vi "ACP Configure Offset Channel.vi"(7 "Selector String":string, 8 "error in (no error)":errorcluster, 10 "ACP Offset Channel Configuration":T1=[{"Offset Frequency"={"Frequency (Hz)"=20000000.0, "Sideband"=2}, "Offset Power Reference"={"Specific Index"=0, "Carrier"=0}, "Integration Bandwidth (Hz)"=18000000.0, "Relative Attenuation (dB)"=0.0, "RRC Filter"={"Alpha"=0.22, "Enabled"=0}, "Enabled"=1}, {"Offset Frequency"={"Frequency (Hz)"=12500000.0, "Sideband"=2}, "Offset Power Reference"={"Specific Index"=0, "Carrier"=0}, "Integration Bandwidth (Hz)"=3840000.0, "Relative Attenuation (dB)"=0.0, "RRC Filter"={"Alpha"=0.22, "Enabled"=0}, "Enabled"=1}, {"Offset Frequency"={"Frequency (Hz)"=17500000.0, "Sideband"=2}, "Offset Power Reference"={"Specific Index"=0, "Carrier"=0}, "Integration Bandwidth (Hz)"=3840000.0, "Relative Attenuation (dB)"=0.0, "RRC Filter"={"Alpha"=0.22, "Enabled"=0}, "Enabled"=1}] {"Enabled" items=["False", "True"]; "Offset Power Reference"."Carrier" items=["Closest", "Highest", "Composite", "Specific"]; "RRC Filter"."Enabled" items=["False", "True"]; "RRC Filter"."Alpha" format="%.3g"; "Relative Attenuation (dB)" format="%.2f"; "Integration Bandwidth (Hz)" format="%.3p"; "Offset Frequency"."Sideband" items=["Neg", "Pos", "Both"]; "Offset Frequency"."Frequency (Hz)" format="%.3p"}, 11 "Instrument Handle In":refnum<k21>) -> (0 "error out":errorcluster, 3 "Instrument Handle Out":refnum<k21>)   [LabVIEW 2016, in "RFmxSpecAn.lvlib"]
uses:
  RFmxSpecAn.lvlib
  Typedefs/ACP Offset Channel Configuration.ctl
  <vilib>/RFmx/SpecAn/mx/RFmxSpecAn.llb/RFmxSpecAn Build Signal String.vi
  <vilib>/RFmx/RFInstr/mx/RFmxInstr.llb/RFmxInstr Build Signal String.vi
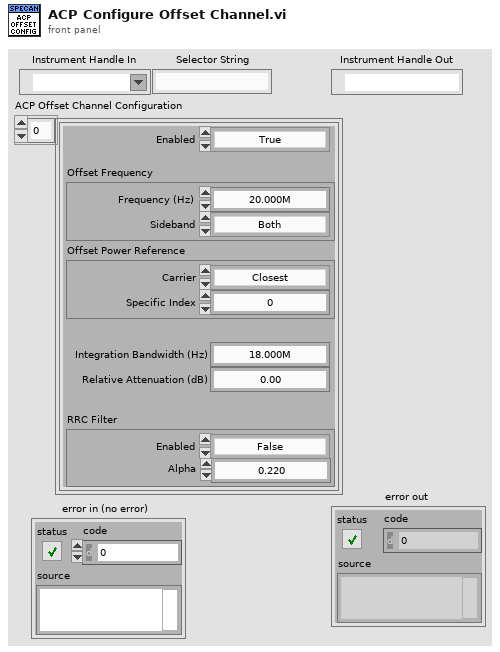
[diagram p1: front panel]
types:
  T1 = typedef "RFmxSpecAn.lvlib/ACP Offset Channel Configuration.ctl" = cluster{"Offset Frequency":cluster{"Frequency (Hz)":dbl, "Sideband":i32}, "Offset Power Reference":cluster{"Specific Index":i32, "Carrier":i32}, "Integration Bandwidth (Hz)":dbl, "Relative Attenuation (dB)":dbl, "RRC Filter":cluster{"Alpha":dbl, "Enabled":i32}, "Enabled":i32}[]
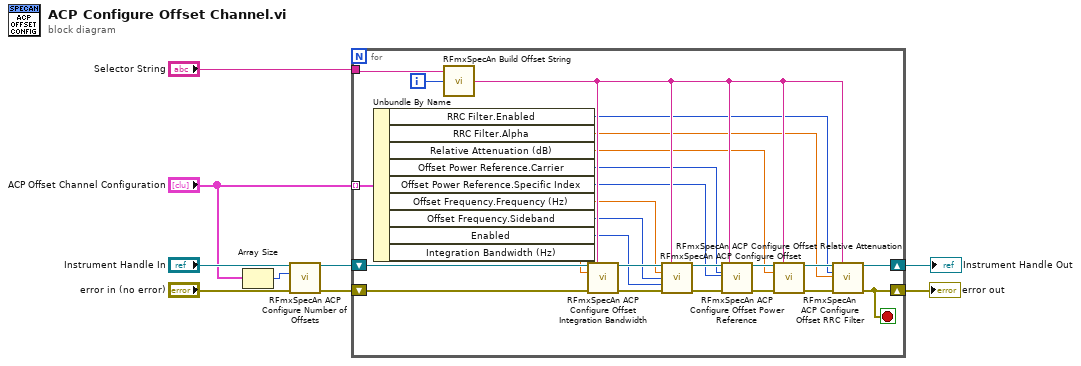
[diagram p0: block diagram]
diagram:
  n1 = Array Size(array="ACP Offset Channel Configuration") -> (size(s)=w7:i32)
  n2 = call <vilib>:"RFmxSpecAn ACP Configure Number of Offsets.vi"("Instrument Handle In"="Instrument Handle In", "Number of Offsets"=w7, "error in (no error)"="error in (no error)") -> ("Instrument Handle Out"=w9:refnum<k21>, "error out"=w8:errorcluster)  [unwired: 11 in]
  n3 = for {
    tunnel: "ACP Offset Channel Configuration" -> [w34] mode=indexing
    shift-right: [w20] -> w5
    shift-left: w8 -> [w32]
    shift-right: [w23] -> w4
    shift-left: w9 -> [w33]
    tunnel: "Selector String" -> [w10]
    i -> [w22]
    stop <- w20 stop-if-true
    n4 = Unbundle By Name(w34) -> ("RRC Filter.Enabled"=w19:i32, "RRC Filter.Alpha"=w18:dbl, "Relative Attenuation (dB)"=w17:dbl, "Offset Power Reference.Carrier"=w16:i32, "Offset Power Reference.Specific Index"=w15:i32, "Offset Frequency.Frequency (Hz)"=w14:dbl, "Offset Frequency.Sideband"=w13:i32, "Enabled"=w12:i32, "Integration Bandwidth (Hz)"=w11:dbl)
    n5 = call <vilib>:"RFmxSpecAn Build Offset String.vi"("Signal Name"=w10, "Offset Number"=w22) -> ("Offset String"=w21:string)  [unwired: 13 in]
    n6 = call <vilib>:"RFmxSpecAn ACP Configure Offset Integration Bandwidth.vi"("Instrument Handle In"=w33, "Selector String"=w21, "Integration Bandwidth (Hz)"=w11, "error in (no error)"=w32) -> ("Instrument Handle Out"=w31:refnum<k21>, "error out"=w30:errorcluster)  [unwired: 10 in]
    n7 = call <vilib>:"RFmxSpecAn ACP Configure Offset.vi"("Instrument Handle In"=w31, "Selector String"=w21, "Offset Frequency (Hz)"=w14, "Offset Sideband"=w13, "Offset Enabled"=w12, "error in (no error)"=w30) -> ("Instrument Handle Out"=w29:refnum<k21>, "error out"=w28:errorcluster)  [unwired: 8 in]
    n8 = call <vilib>:"RFmxSpecAn ACP Configure Offset Power Reference.vi"("Instrument Handle In"=w29, "Selector String"=w21, "Offset Power Reference Carrier"=w16, "Offset Power Reference Specific"=w15, "error in (no error)"=w28) -> ("Instrument Handle Out"=w27:refnum<k21>, "error out"=w26:errorcluster)  [unwired: 9 in]
    n9 = call <vilib>:"RFmxSpecAn ACP Configure Offset Relative Attenuation.vi"("Instrument Handle In"=w27, "Selector String"=w21, "Relative Attenuation (dB)"=w17, "error in (no error)"=w26) -> ("Instrument Handle Out"=w25:refnum<k21>, "error out"=w24:errorcluster)  [unwired: 10 in]
    n10 = call <vilib>:"RFmxSpecAn ACP Configure Offset RRC Filter.vi"("Instrument Handle In"=w25, "Selector String"=w21, "RRC Filter Enabled"=w19, "RRC Alpha"=w18, "error in (no error)"=w24) -> ("Instrument Handle Out"=w23:refnum<k21>, "error out"=w20:errorcluster)  [unwired: 9 in]
  }
  "Instrument Handle Out" <- w4
  "error out" <- w5
